vi "Init Module.vi"(8 "error in (no error)":errorcluster, 11 "OtherModule in":refnum<class "OtherModule.lvclass">) -> (0 "error out":errorcluster, 3 "OtherModule out":refnum<class "OtherModule.lvclass">)   [LabVIEW 2020, in "VolatusScratch.lvlib" / "OtherModule.lvclass"]
uses:
  OtherModule.lvclass
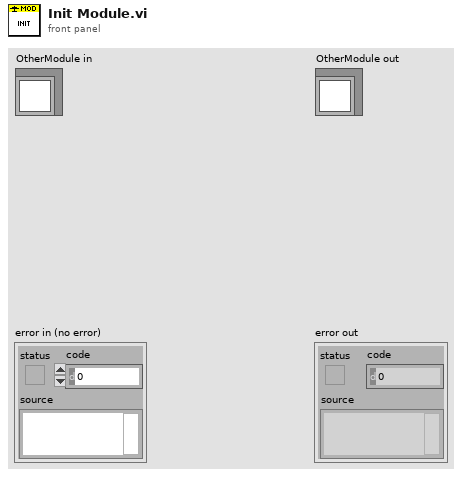
[diagram p1: front panel]
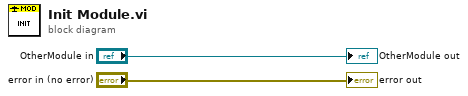
[diagram p0: block diagram]
diagram:
  "error out" <- "error in (no error)"
  "OtherModule out" <- "OtherModule in"
